vi "Get Slope.vi"(8 "error in (no error)":errorcluster, 11 "VISA resource name":refnum<visa-resource-name>) -> (0 "error out":errorcluster, 2 "Filter Slope":T1, 3 "VISA resource name out":refnum<visa-resource-name>)   [LabVIEW 2016, in "SR7270 Drivers.lvclass"]
uses:
  SR7270 Drivers.lvclass
  Typedefs/SLOPE--enum.ctl
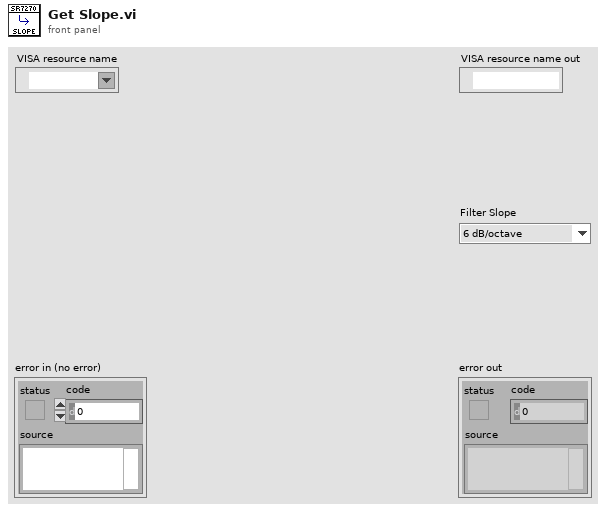
[diagram p1: front panel]
types:
  T1 = typedef "SR7270 Drivers.lvclass/SLOPE--enum.ctl" = enum16{"6 dB/octave", "12 dB/octave", "18 dB/octave", "24 dB/octave"}
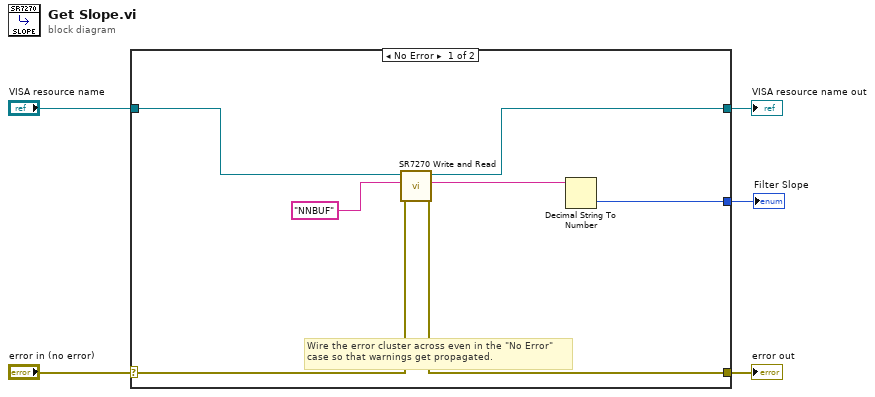
[diagram p0: block diagram]
diagram:
  n1 = case shown="No Error" "error in (no error)" {
    selector: "error in (no error)" -> [w12 w14]
    tunnel: [w11 w14] -> w4
    tunnel: [w7 w13] -> w2
    tunnel: "VISA resource name" -> [w6 w13]
    tunnel: [w8 _] -> w1
    frame No Error {
      # "Wire the error cluster across even in the \"No Error\"\ncase so that warnings get propagated."
      n2 = call "SR7270 Write and Read.vi"("error in (no error)"=w12, "Command Name"="NNBUF", "VISA resource name"=w6) -> ("error out"=w11:errorcluster, "Read"=w9:string, "VISA resource name out"=w7:refnum<visa-resource-name>)  [unwired: 5 in, 1 out]
      n3 = Decimal String To Number(string=w9) -> (number=w8:i32)  [unwired: 2 in, 1 out]
    }
    frame Error {
    }
  }
  "error out" <- w4
  "VISA resource name out" <- w2
  "Filter Slope" <- w1
